vi "midiPlayer.announcements.get.vi"(11 "midiPlayer":refnum<class "midiPlayer.lvclass">) -> (2 "midiPlayer.Announcements":refnum<user-event>)   [LabVIEW 2020, in "midiPlayer.lvclass"]
uses:
  midiPlayer.lvclass
  midiPlayer.lvclass/midiPlayer.ctl
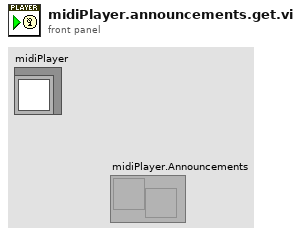
[diagram p1: front panel]
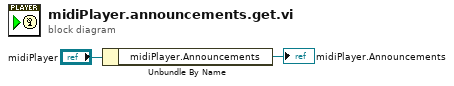
[diagram p0: block diagram]
diagram:
  n1 = Unbundle By Name("midiPlayer") -> ("midiPlayer.Announcements"=→"midiPlayer.Announcements":refnum<user-event>)
